vi "Actor Core.vi"(8 "error in":errorcluster, 11 "CS++GoBangClient in":refnum<class "CS++GoBangClient.lvclass">) -> (0 "error out":errorcluster, 3 "Actor out":refnum<class "Actor.lvclass">)   [LabVIEW 2014, in "GoBang.lvlib" / "CS++GoBangClient.lvclass"]
doc: "(<B>Filename</B>: Actor Framework.lvlib:Actor.lvclass:Actor Core.vi)\n\nReceives messages to the actor, reacts to them, and initiates any error handling that may shut the actor down.\n\nDescendant classes may override this VI to append parallel tasks for the actor to complete while it handles messages. Overrides use the Call Parent Method node."
uses:
  CS++GoBangClient.lvclass
  <vilib>/ActorFramework/Actor/Actor.lvclass
  typdefs/BoardField.ctl
  typdefs/GameState.ctl
  CSPP_Core/Actors/CS++SVMonitor/CS++SVMonitor.lvclass
  CS++GoBangClient Messages/Write black player Msg/Write black player Msg.lvclass
  CS++GoBangClient Messages/Write white player Msg/Write white player Msg.lvclass
  CS++GoBangClient Messages/Write game board Msg/Write game board Msg.lvclass
  CS++GoBangClient Messages/Write game state Msg/Write game state Msg.lvclass
  CSPP_Core/Actors/CS++BaseActor/CS++BaseActor.lvclass/CS++BaseActor.ctl
  <vilib>/ActorFramework/Actor/Actor.lvclass/Actor.ctl
  <vilib>/ActorFramework/Message Enqueuer/Message Enqueuer.lvclass/Message Enqueuer.ctl
  CS++GoBangClient.lvclass/CS++GoBangClient.ctl
  CSPP_Core/Actors/CS++PVMonitor Messages/Register PVs Msg/Register PVs Msg.lvclass/Register PVs Msg.ctl
  CS++GoBangClient Messages/Send Move Msg/Send Move Msg.lvclass/Send Move Msg.ctl
  CS++GoBangClient Messages/Join Game Msg/Join Game Msg.lvclass/Join Game Msg.ctl
  <vilib>/ActorFramework/Message Enqueuer/Init from Existing Queue.vi
  <vilib>/ActorFramework/Message Enqueuer/Enqueue.vi
  <vilib>/ActorFramework/Message Priority Queue/Priority Enqueue.vi
  <vilib>/ActorFramework/Message Enqueuer/Message Enqueuer.lvclass
  CSPP_Core/Actors/CS++PVMonitor Messages/Register PVs Msg/Register PVs Msg.lvclass
  CS++GoBangClient Messages/Send Move Msg/Send Move Msg.lvclass
  CS++GoBangClient Messages/Join Game Msg/Join Game Msg.lvclass
  <vilib>/ActorFramework/Stop Msg/Stop Msg.lvclass
  CSPP_Core/Actors/CS++BaseActor/CS++BaseActor.lvclass
  GoBang.lvlib
  CSPP_Core/Classes/CS++ProcessVariables/PVConnection/PVConnection.lvclass
panel:
  in  "OppColor":T1
  out "Opponnents name":string
  in  "Color":T1
  in  "Your name":string
  in  "stone":T1
  in  "stop":bool
  in  "State":T2
  out "GameBoard":T1[][](array[typedef])
  out "White won":bool
  out "Black won":bool
  out "Game over":bool
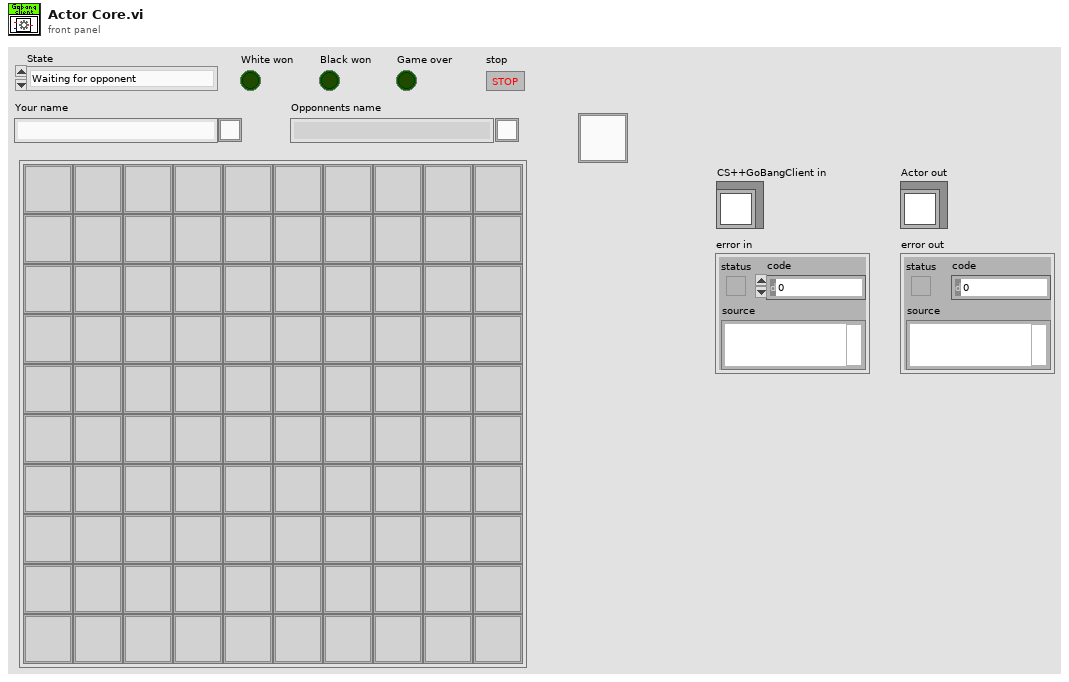
[diagram p1: front panel]
types:
  T1 = typedef "GoBang.lvlib/BoardField.ctl" = u8
  T2 = typedef "GoBang.lvlib/GameState.ctl" = enum16{"Waiting for opponent", "White to move", "Black to move", "Game over, white won", "Game over, black won"}
  T3 = enum32{"Invalid", "Standard", "Closed", "Hidden", "Minimized", "Maximized"}
  T4 = cluster{"BlackPlayer":string, "GoBang.lvlib:Write black player Msg.lvclass":refnum<class "Write black player Msg.lvclass">}
  T5 = cluster{"GameBoard":string, "GoBang.lvlib:Write game board Msg.lvclass":refnum<class "Write game board Msg.lvclass">}
  T6 = cluster{"GameState":string, "GoBang.lvlib:Write game state Msg.lvclass":refnum<class "Write game state Msg.lvclass">}
  T7 = cluster{"WhitePlayer":string, "GoBang.lvlib:Write white player Msg.lvclass":refnum<class "Write white player Msg.lvclass">}
  T8 = cluster{"GameState":string, "GoBang.lvlib:Write white player Msg.lvclass":refnum<class "CS++PVUpdate Msg.lvclass">}[]
  T9 = cluster{"Self Enqueuer":refnum<class "Message Enqueuer.lvclass">, cluster{"GameState":string, "GoBang.lvlib:Write white player Msg.lvclass":refnum<class "CS++PVUpdate Msg.lvclass">}[]}
  T10 = typedef "LVPositionTypeDef.ctl" = cluster{"Left":i32, "Top":i32}
  T11 = typedef "LVBoundsTypeDef.ctl" = cluster{"Width":u32, "Height":u32}
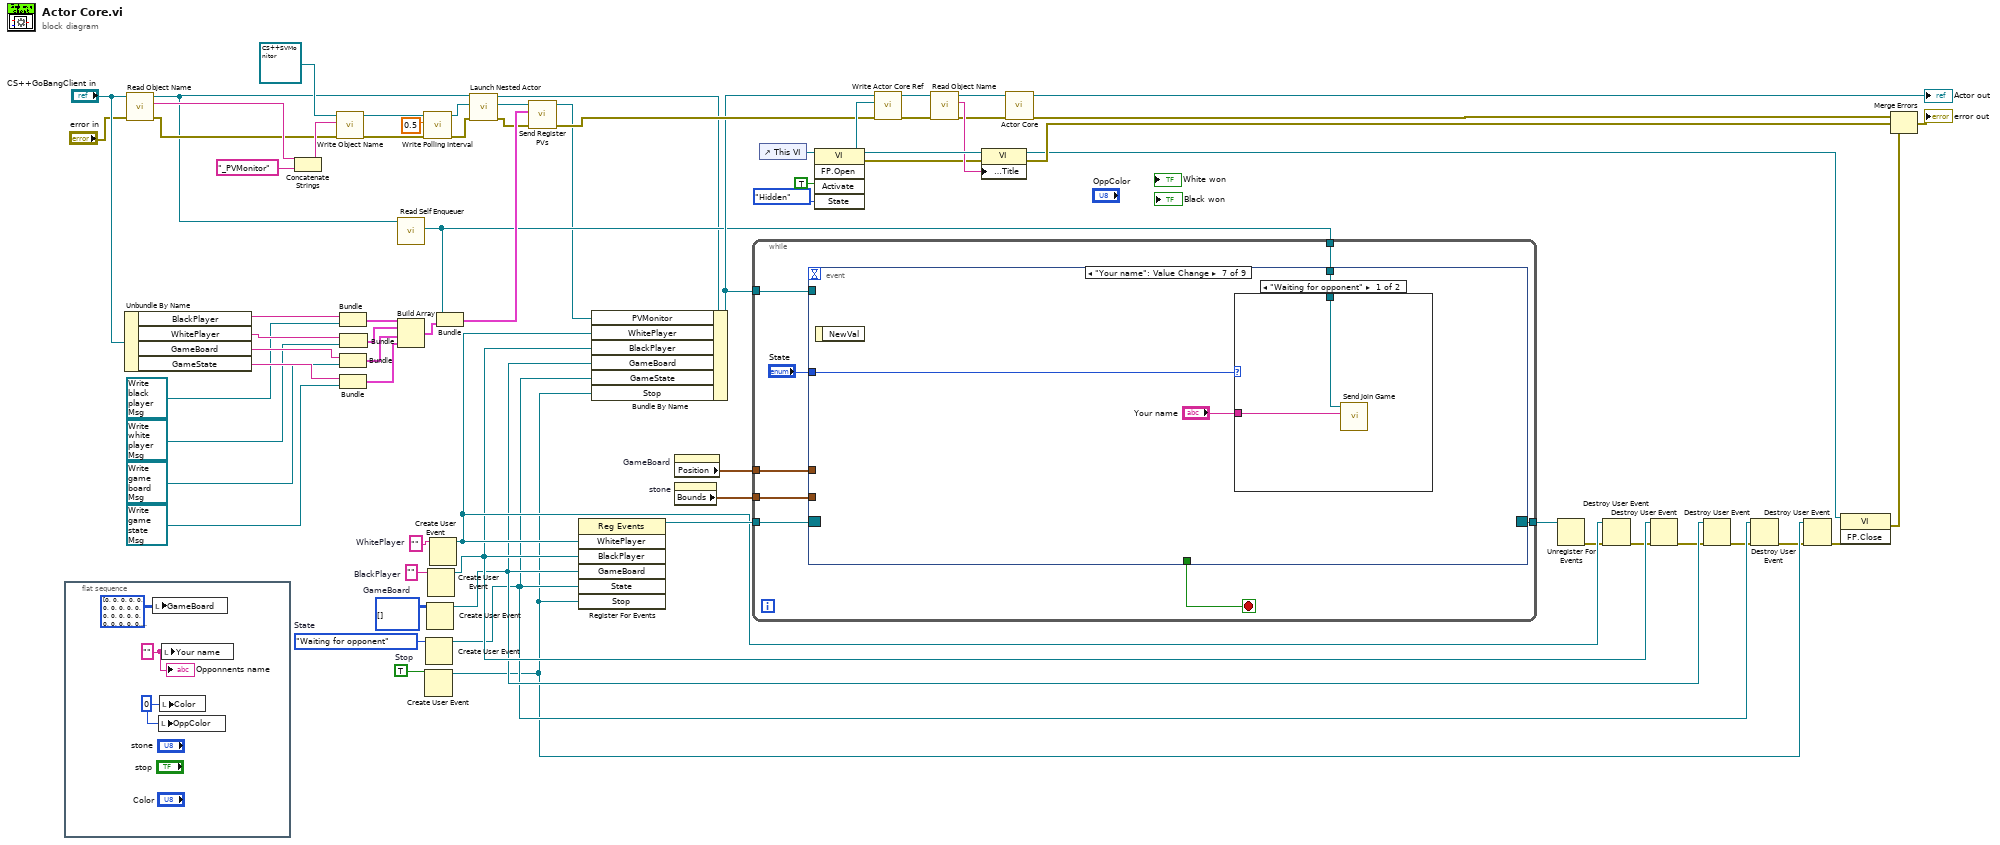
[diagram p0: block diagram]
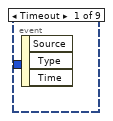
[diagram p2: hidden frame]
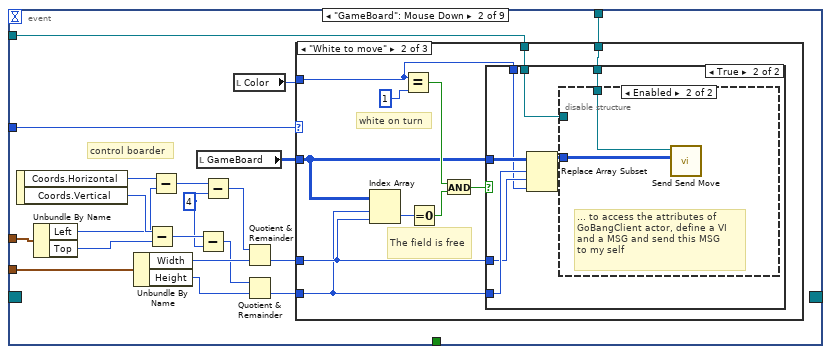
[diagram p3: hidden frame]
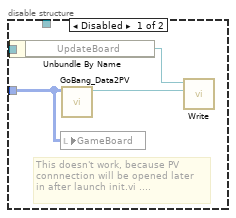
[diagram p6: hidden frame]
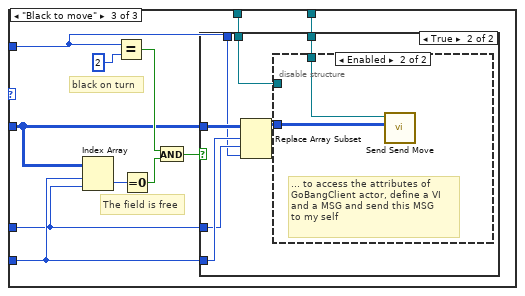
[diagram p7: hidden frame]
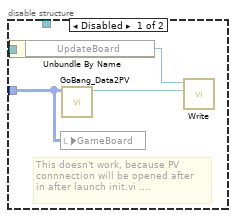
[diagram p9: hidden frame]
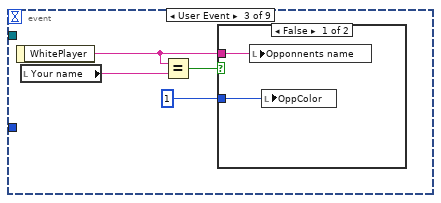
[diagram p10: hidden frame]
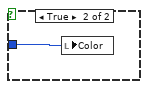
[diagram p11: hidden frame]
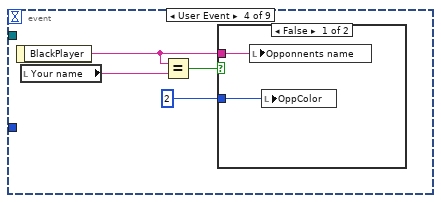
[diagram p12: hidden frame]
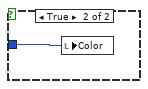
[diagram p13: hidden frame]
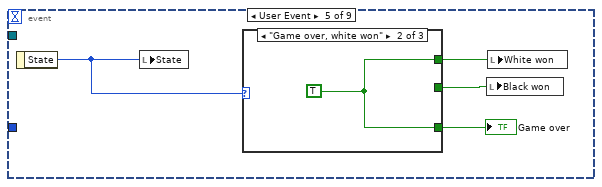
[diagram p14: hidden frame]
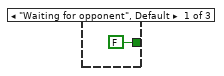
[diagram p15: hidden frame]
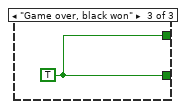
[diagram p16: hidden frame]
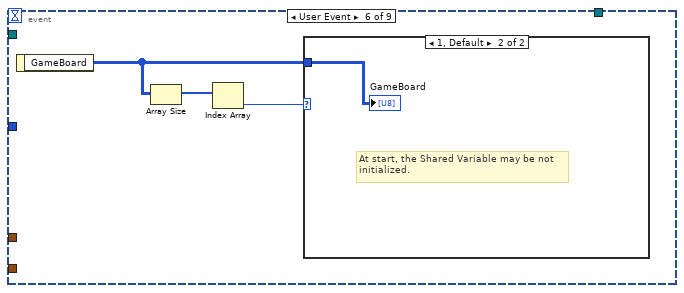
[diagram p17: hidden frame]
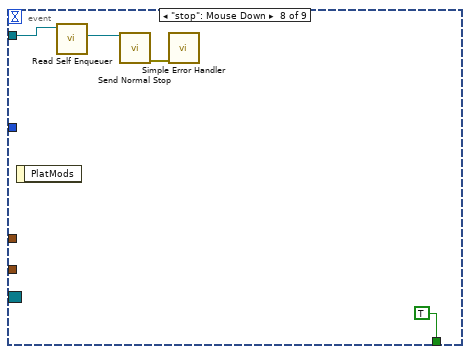
[diagram p20: hidden frame]
diagram:
  w41 = TRUE  # Stop
  w47 = T1[][] []  # GameBoard
  w48 = GameState."Waiting for opponent"  # State
  w49 = ""  # BlackPlayer
  w50 = ""  # WhitePlayer
  n1 = flat-sequence {
    frame #0 {
      w71 = T1 0 ("Color")
      w70 = "" ("Your name")
      n2 = local write "GameBoard"(T1[][] [[0, 0, 0, 0, 0, 0, 0, 0, 0, 0], [0, 0, 0, 0, 0, 0, 0, 0, 0, 0], [0, 0, 0, 0, 0, 0, 0, 0, 0, 0], [0, 0, 0, 0, 0, 0, 0, 0, 0, 0], [0, 0, 0, 0, 0, 0, 0, 0, 0, 0], [0, 0, 0, 0, 0, 0, 0, 0, 0, 0], [0, 0, 0, 0, 0, 0, 0, 0, 0, 0], [0, 0, 0, 0, 0, 0, 0, 0, 0, 0], [0, 0, 0, 0, 0, 0, 0, 0, 0, 0], [0, 0, 0, 0, 0, 0, 0, 0, 0, 0]] ("GameBoard")) -> ()
      n3 = local write "OppColor"(w71) -> ()
      n4 = local write "Color"(w71) -> ()
      n5 = local write "Your name"(w70) -> ()
      "Opponnents name" <- w70
    }
  }
  n6 = Unbundle By Name("CS++GoBangClient in") -> ("BlackPlayer"=w65:string, "WhitePlayer"=w56:string, "GameBoard"=w55:string, "GameState"=w54:string)
  n7 = call "Read Object Name.vi"("error in (no error)"="error in", "CS++BaseActor in"="CS++GoBangClient in") -> ("error out"=w28:errorcluster, "Object Name"=w58:string, "CS++BaseActor out"=w9:refnum<class "CS++GoBangClient.lvclass">)  [unwired: 7 in]
  n8 = Concatenate Strings(w58, "_PVMonitor" ("Object Name")) -> (w61:string)
  n9 = call "Write Object Name.vi"("error in (no error)"=w28, "Object Name"=w61, "CS++BaseActor in"=refnum<class "CS++SVMonitor.lvclass"> refnum ("CS++SVMonitor.lvlib:CS++SVMonitor.lvclass")) -> ("error out"=w3:errorcluster, "CS++BaseActor out"=w5:refnum<class "CS++SVMonitor.lvclass">)  [unwired: 7 in]
  n10 = Bundle("BlackPlayer"=w65, "GoBang.lvlib:Write black player Msg.lvclass"=refnum<class "Write black player Msg.lvclass"> refnum) -> (w64:T4)  [unwired: 1 in]
  n11 = Bundle("GameBoard"=w55, "GoBang.lvlib:Write game board Msg.lvclass"=refnum<class "Write game board Msg.lvclass"> refnum) -> (w52:T5)  [unwired: 1 in]
  n12 = Bundle("GameState"=w54, "GoBang.lvlib:Write game state Msg.lvclass"=refnum<class "Write game state Msg.lvclass"> refnum) -> (w51:T6)  [unwired: 1 in]
  n13 = Bundle("WhitePlayer"=w56, "GoBang.lvlib:Write white player Msg.lvclass"=refnum<class "Write white player Msg.lvclass"> refnum) -> (w53:T7)  [unwired: 1 in]
  n14 = call <vilib>:"Read Self Enqueuer.vi"("Actor"=w9) -> ("Self Enqueuer"=w14:refnum<class "Message Enqueuer.lvclass">)  [unwired: 10 in]
  n15 = Build Array(w64, w53, w52, w51) -> (w63:T8)
  n16 = call "Write Polling Interval.vi"("error in (no error)"=w3, "Polling Interval"=dbl[unit] 0.5 ("Interval"), "CS++BaseActor in"=w5) -> ("error out"=w2:errorcluster, "CS++BaseActor out"=w1:refnum<class "CS++SVMonitor.lvclass">)  [unwired: 7 in]
  n17 = Create User Event(user event datatype=w41) -> (user event=w21:refnum<user-event>)  [unwired: 1 in, 1 out]
  n18 = Create User Event(user event datatype=w48) -> (user event=w22:refnum<user-event>)  [unwired: 1 in, 1 out]
  n19 = Create User Event(user event datatype=w47) -> (user event=w23:refnum<user-event>)  [unwired: 1 in, 1 out]
  n20 = Create User Event(user event datatype=w49) -> (user event=w24:refnum<user-event>)  [unwired: 1 in, 1 out]
  n21 = Create User Event(user event datatype=w50) -> (user event=w25:refnum<user-event>)  [unwired: 1 in, 1 out]
  n22 = Bundle("Self Enqueuer"=w14, w63) -> (w59:T9)  [unwired: 1 in]
  n23 = call <vilib>:"Launch Nested Actor.vi"("error in (no error)"=w2, "Nested Actor"=w1, "Caller Actor in"=w9) -> ("error out"=w6:errorcluster, "Nested Actor's Enqueuer"=w7:refnum<class "Message Enqueuer.lvclass">, "Caller Actor out"=w8:refnum<class "CS++GoBangClient.lvclass">)  [unwired: 6 in]
  n24 = call "Send Register PVs.vi"("error in (no error)"=w6, "Register Info"=w59, "Message Enqueuer"=w7) -> ("error out"=w27:errorcluster)  [unwired: 7 in, 1 out]
  n25 = register-events(w25, w24, w23, w22, w21) -> (reference out=w46:refnum<event-registration>)  [unwired: 2 in, 1 out]
  n26 = Bundle By Name(cluster=w8, "PVMonitor"=w7, "WhitePlayer"=w25, "BlackPlayer"=w24, "GameBoard"=w23, "GameState"=w22, "Stop"=w21) -> (w15:refnum<class "CS++GoBangClient.lvclass">)
  n27 = property on="GameBoard" class="Arr (strict)"() -> ("Position"=w66:T10)  [unwired: 2 in, 2 out]
  n28 = property on="stone" class="Ring (strict)"() -> ("Bounds"=w67:T11)  [unwired: 2 in, 2 out]
  n29 = while {
    tunnel: w67 -> [w79]
    tunnel: w66 -> [w78]
    tunnel: w46 -> [w77]
    tunnel: w15 -> [w76]
    tunnel: [w74] -> w26
    tunnel: w14 -> [w73]
    stop <- w80 stop-if-true
    n30 = event shown="[6] \"Your name\": Value Change" {
      selector: w77 -> [_ _ _ _ _ _ _ _ _]
      dyn-events: [_ _ _ _ _ _ _ _ _] -> w74
      timeout: _ -> [_ _ _ _ _ _ _ _ _]
      tunnel: [_ _ _ _ _ _ _ TRUE TRUE] -> w80
      tunnel: w79 -> [_ w100 _ _ _ _ _ _ _]
      tunnel: w78 -> [_ w95 _ _ _ _ _ _ _]
      tunnel: w76 -> [_ w82 _ _ _ _ _ w181 _]
      tunnel: "State" -> [_ w85 _ _ _ _ w176 _ _]
      tunnel: w73 -> [_ w81 _ _ _ _ w174 _ _]
      event Timeout {
        n31 = event-data() -> ()  [unwired: 1 in, 3 out]
      }
      event "GameBoard": Mouse Down {
        w88 = 4 ("y 2")
        # "control boarder"
        n32 = event-data() -> ("Coords.Horizontal"=w99:i32, "Coords.Vertical"=w97:i32)  [unwired: 1 in]
        n33 = Unbundle By Name(w95) -> ("Left"=w94:i32, "Top"=w93:i32)
        n34 = Unbundle By Name(w100) -> ("Width"=w98:u32, "Height"=w96:u32)
        n35 = Subtract(x=w97, y=w93) -> (x-y=w91:i32)
        n36 = Subtract(x=w99, y=w94) -> (x-y=w92:i32)
        n37 = local read "GameBoard"() -> (w84:T1[][])
        n38 = Subtract(x=w91, y=w88) -> (x-y=w89:i32)
        n39 = Subtract(x=w92, y=w88) -> (x-y=w90:i32)
        n40 = local read "Color"() -> (w83:T1)
        n41 = Quotient & Remainder(x=w90, y=w98) -> (floor(x/y)=w87:u32)  [unwired: 1 out]
        n42 = Quotient & Remainder(x=w89, y=w96) -> (floor(x/y)=w86:u32)  [unwired: 1 out]
        n43 = case shown="\"White to move\"" w85 {
          tunnel: w87 -> [_ w103 w134]
          tunnel: w86 -> [_ w102 w135]
          tunnel: w84 -> [_ w105 w129]
          tunnel: w83 -> [_ w101 w127]
          tunnel: w82 -> [_ w106 w126]
          tunnel: w81 -> [_ w107 w125]
          frame "Waiting for opponent", Default {
          }
          frame "White to move" {
            # "white on turn"
            # "The field is free"
            n44 = Index Array(array=w105, index (row)=w102, index (col)=w103) -> (element=w111:T1)
            n45 = Equal?(x=w101, y=T1 1) -> (x = y?=w109:bool)
            n46 = Equal To 0?(x=w111) -> (x = 0?=w110:bool)
            n47 = And(x=w109, y=w110) -> (x .and. y?=w104:bool)
            n48 = case shown="True" w104 {
              tunnel: w102 -> [_ w118]
              tunnel: w103 -> [_ w117]
              tunnel: w105 -> [_ w116]
              tunnel: w101 -> [_ w115]
              tunnel: w106 -> [_ w113]
              tunnel: w107 -> [_ w112]
              frame False {
              }
              frame True {
                n49 = Replace Array Subset(array=w116, new element=w115, index (row)=w118, index (col)=w117) -> (w114:T1[][])
                n50 = disable-structure shown="Enabled" {
                  disable-tunnel: w114 -> [w121 w123]
                  disable-tunnel: w113 -> [w119 _]
                  disable-tunnel: w112 -> [_ w124]
                  frame Disabled {
                    # "This doesn't work, because PV\nconnnection will be opened later\nin after launch init.vi ...."
                    n51 = Unbundle By Name(w119) -> ("UpdateBoard"=w120:refnum<class "PVConnection.lvclass">)
                    n52 = local write "GameBoard"(w121) -> ()
                    n53 = call "GoBang_Data2PV.vi"("Data in"=w121) -> ("PV out"=w122:refnum<class "PV.lvclass">)  [unwired: 10 in]
                    n54 = call "Write.vi"("PV"=w122, "PVConnection in"=w120) -> ()  [unwired: 8 in, 2 out]
                  }
                  frame Enabled {
                    # "... to access the attributes of \nGoBangClient actor, define a VI \nand a MSG and send this MSG \nto my self"
                    n55 = call "Send Send Move.vi"("GameBoard"=w123, "Message Enqueuer"=w124) -> ()  [unwired: 8 in, 2 out]
                  }
                }
              }
            }
          }
          frame "Black to move" {
            # "black on turn"
            # "The field is free"
            n56 = Index Array(array=w129, index (row)=w135, index (col)=w134) -> (element=w133:T1)
            n57 = Equal?(x=w127, y=T1 2) -> (x = y?=w130:bool)
            n58 = Equal To 0?(x=w133) -> (x = 0?=w131:bool)
            n59 = And(x=w130, y=w131) -> (x .and. y?=w132:bool)
            n60 = case shown="True" w132 {
              tunnel: w135 -> [_ w142]
              tunnel: w134 -> [_ w141]
              tunnel: w129 -> [_ w140]
              tunnel: w127 -> [_ w139]
              tunnel: w126 -> [_ w137]
              tunnel: w125 -> [_ w136]
              frame False {
              }
              frame True {
                n61 = Replace Array Subset(array=w140, new element=w139, index (row)=w142, index (col)=w141) -> (w138:T1[][])
                n62 = disable-structure shown="Enabled" {
                  disable-tunnel: w138 -> [w145 w147]
                  disable-tunnel: w137 -> [w143 _]
                  disable-tunnel: w136 -> [_ w148]
                  frame Disabled {
                    # "This doesn't work, because PV\nconnnection will be opened after\nin after launch init.vi ...."
                    n63 = Unbundle By Name(w143) -> ("UpdateBoard"=w144:refnum<class "PVConnection.lvclass">)
                    n64 = local write "GameBoard"(w145) -> ()
                    n65 = call "GoBang_Data2PV.vi"("Data in"=w145) -> ("PV out"=w146:refnum<class "PV.lvclass">)  [unwired: 10 in]
                    n66 = call "Write.vi"("PV"=w146, "PVConnection in"=w144) -> ()  [unwired: 8 in, 2 out]
                  }
                  frame Enabled {
                    # "... to access the attributes of \nGoBangClient actor, define a VI \nand a MSG and send this MSG \nto my self"
                    n67 = call "Send Send Move.vi"("GameBoard"=w147, "Message Enqueuer"=w148) -> ()  [unwired: 8 in, 2 out]
                  }
                }
              }
            }
          }
        }
      }
      event User Event {
        n68 = event-data() -> ("WhitePlayer"=w150:string)  [unwired: 1 in]
        n69 = local read "Your name"() -> (w152:string)
        n70 = Equal?(x=w150, y=w152) -> (x = y?=w151:bool)
        n71 = case shown="False" w151 {
          tunnel: w150 -> [w154 _]
          tunnel: T1 1 ("Color") -> [w153 w155]
          frame False {
            n72 = local write "Opponnents name"(w154) -> ()
            n73 = local write "OppColor"(w153) -> ()
          }
          frame True {
            n74 = local write "Color"(w155) -> ()
          }
        }
      }
      event User Event {
        n75 = event-data() -> ("BlackPlayer"=w157:string)  [unwired: 1 in]
        n76 = local read "Your name"() -> (w159:string)
        n77 = Equal?(x=w157, y=w159) -> (x = y?=w158:bool)
        n78 = case shown="False" w158 {
          tunnel: w157 -> [w161 _]
          tunnel: T1 2 ("Color") -> [w160 w162]
          frame False {
            n79 = local write "Opponnents name"(w161) -> ()
            n80 = local write "OppColor"(w160) -> ()
          }
          frame True {
            n81 = local write "Color"(w162) -> ()
          }
        }
      }
      event User Event {
        n82 = event-data() -> ("State"=w166:T2)  [unwired: 1 in]
        n83 = local write "State"(w166) -> ()
        n84 = case shown="\"Game over, white won\"" w166 {
          tunnel: [FALSE ("White won") w168 w169] -> w165
          tunnel: [_ _ w169] -> w164
          tunnel: [_ w168 _] -> w163
          frame "Waiting for opponent", Default {
          }
          frame "Game over, white won" {
            w168 = TRUE ("White won")
          }
          frame "Game over, black won" {
            w169 = TRUE ("White won")
          }
        }
        "Game over" <- w165
        n85 = local write "Black won"(w164) -> ()
        n86 = local write "White won"(w163) -> ()
      }
      event User Event {
        n87 = event-data() -> ("GameBoard"=w170:T1[][])  [unwired: 1 in]
        n88 = Array Size(array=w170) -> (size(s)=w172:i32[])
        n89 = Index Array(array=w172) -> (element=w171:i32)  [unwired: 1 in]
        n90 = case shown="1, Default" w171 {
          tunnel: w170 -> [_ w173]
          frame 0 {
          }
          frame 1, Default {
            # "At start, the Shared Variable may be not\ninitialized."
            "GameBoard" <- w173
          }
        }
      }
      event "Your name": Value Change {
        n91 = event-data() -> ()  [unwired: 1 in, 1 out]
        n92 = case shown="\"Waiting for opponent\"" w176 {
          tunnel: "Your name" -> [w177 _]
          tunnel: w174 -> [w178 _]
          frame "Waiting for opponent" {
            n93 = call "Send Join Game.vi"("Your name"=w177, "Message Enqueuer"=w178) -> ()  [unwired: 8 in, 2 out]
          }
          frame "White to move", Default {
          }
        }
      }
      event "stop": Mouse Down {
        n94 = event-data() -> ()  [unwired: 1 in, 1 out]
        n95 = call <vilib>:"Read Self Enqueuer.vi"("Actor"=w181) -> ("Self Enqueuer"=w179:refnum<class "Message Enqueuer.lvclass">)  [unwired: 10 in]
        n96 = call <vilib>:"Send Normal Stop.vi"("Message Enqueuer"=w179) -> ("error out"=w180:errorcluster)  [unwired: 10 in]
        n97 = call <vilib>:"Simple Error Handler.vi"("error in (no error)"=w180) -> ()  [unwired: 4 in, 5 out]
      }
      event User Event {
        n98 = event-data() -> ()  [unwired: 1 in, 5 out]
      }
    }
  }
  n99 = control-ref of="This VI"() -> (w38:refnum<vi>)
  n100 = invoke class="VI" method="FP.Open"(reference=w38, "Activate"=TRUE ("Activate?"), "State"=T3."Hidden") -> (reference out=w35:refnum<vi>, error out=w30:errorcluster)  [unwired: 2 in, 3 out]
  n101 = call "Write Actor Core Ref.vi"("error in (no error)"=w27, "Actor Core Ref"=w35, "CS++BaseActor in"=w15) -> ("error out"=w36:errorcluster, "CS++BaseActor out"=w37:refnum<class "CS++GoBangClient.lvclass">)  [unwired: 7 in]
  n102 = call "Read Object Name.vi"("error in (no error)"=w36, "CS++BaseActor in"=w37) -> ("error out"=w32:errorcluster, "Object Name"=w34:string, "CS++BaseActor out"=w33:refnum<class "CS++GoBangClient.lvclass">)  [unwired: 7 in]
  n103 = property class="VI"(reference=w35, error in=w30, "Front Panel.Title"=w34) -> (reference out=w12:refnum<vi>, error out=w29:errorcluster)
  n104 = call-parent "Actor Core.vi"("error in"=w32, "CS++BaseActor in"=w33) -> ("error out"=w69:errorcluster, "Actor out"=→"Actor out":refnum<class "Actor.lvclass">)  [unwired: 8 in]
  n105 = Unregister For Events(event registration refnum=w26) -> (error out=w20:errorcluster)  [unwired: 1 in]
  n106 = Destroy User Event(user event=w25, error in=w20) -> (error out=w19:errorcluster)
  n107 = Destroy User Event(user event=w24, error in=w19) -> (error out=w18:errorcluster)
  n108 = Destroy User Event(user event=w23, error in=w18) -> (error out=w17:errorcluster)
  n109 = Destroy User Event(user event=w22, error in=w17) -> (error out=w16:errorcluster)
  n110 = Destroy User Event(user event=w21, error in=w16) -> (error out=w13:errorcluster)
  n111 = invoke class="VI" method="FP.Close"(reference=w12, error in=w13) -> (error out=w10:errorcluster)  [unwired: 1 in, 2 out]
  n112 = Merge Errors(w69, w29, w10) -> (→"error out":errorcluster)
